vi "tank_auto_sub_straight.vi"(8 "Input Data":i32[](array[numeric]), 10 "Drive Control":T2={"Left X"=0, "Left Y"=0, "Right Y"=0, "Power (100)"=100, "Wait (ms)"=100, "Enc/Deg Target"=0, "Move Type"=enum."Wait"} {"Power (100)" min=-100 max=100}, 11 "NXT/EV3":T1) -> (0 "Output Data":i32[](array[numeric]), 3 "NXT/EV3 out":T1, 4 "Time Out?":bool)   [LabVIEW 2012, in "Serenity_mk2.lvrbt"]
uses:
  Serenity_mk2.lvrbt
  SubVIs/auto_drive_TYP.ctl
  <vilib>/NXT/Subs/LVHSConnector.ctl
  <vilib>/NXT/LegoClasses/BrickReference/BrickReference.lvclass
  <vilib>/FTC/FTC ControllerState.ctl
  <vilib>/FTC/FTC POVState.ctl
  <vilib>/NXT/Hardware/Plugins/Tetrix DC Motor/TetrixDCMotorAddress.ctl
  <vilib>/NXT/HiTechnic/HiTechnic Controls/HiTechnic Port.ctl
  <vilib>/NXT/Block Support/NXT_InputPort.ctl
  <vilib>/FTC/FTC Calculate Drive Power - Tank.vi
  <vilib>/NXT/NXTIO Xnodes/NXTIONodeSubVIs/TETRIX IO Move DC Motors.vi
  <vilib>/NXT/NXTIO Xnodes/NXTIONodeSubVIs/TETRIX IO Motor Status.vi
  <vilib>/NXT/Dual Mode Library/prims/inRangeAndCoerce/inRangeAndCoerce_int8.vi
  <vilib>/NXT/Dual Mode Library/Sound/Tone.vi
  <vilib>/NXT/NXTIO Xnodes/NXTIONodeSubVIs/TETRIX IO Stop DC Motors.vi
  <vilib>/NXT/NXTIO Xnodes/AddressXNode/NXTIOAddress.xnode
  <vilib>/NXT/NXTIO Xnodes/NXTIOXNode/NXTIO.xnode
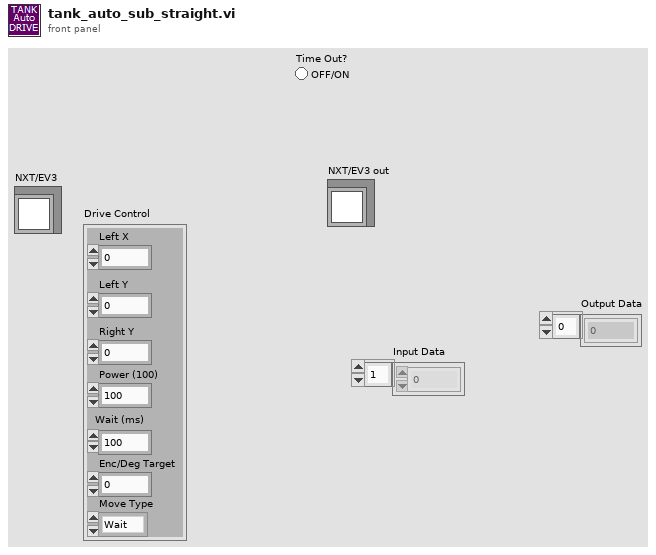
[diagram p1: front panel]
types:
  T1 = typedef "LVHSConnector.ctl" = refnum<class "BrickReference.lvclass">
  T2 = typedef "auto_drive_TYP.ctl" = cluster{"Left X":i8, "Left Y":i8, "Right Y":i8, "Power (100)":i8, "Wait (ms)":u32, "Enc/Deg Target":i32, "Move Type":enum16{"Relative Degrees", "Wait", "Encoder"}}
  T3 = typedef "FTC ControllerState.ctl" = cluster{"Left X":i8, "Left Y":i8, "Right X":i8, "Right Y":i8, "Button Encoding 9-12":u8, "Button Encoding 1-8":u8, "POV":T4}
  T4 = typedef "FTC POVState.ctl" = i8
  T5 = typedef "HiTechnic Port.ctl" = cluster{"Port":T6, "MUX Port":u8}
  T6 = typedef "NXT_InputPort.ctl" = u32
  T7 = typedef "TetrixDCMotorAddress.ctl" = i32
  T8 = cluster{"TetrixDCMotor":T7, "TetrixDCMotor 2":T7}
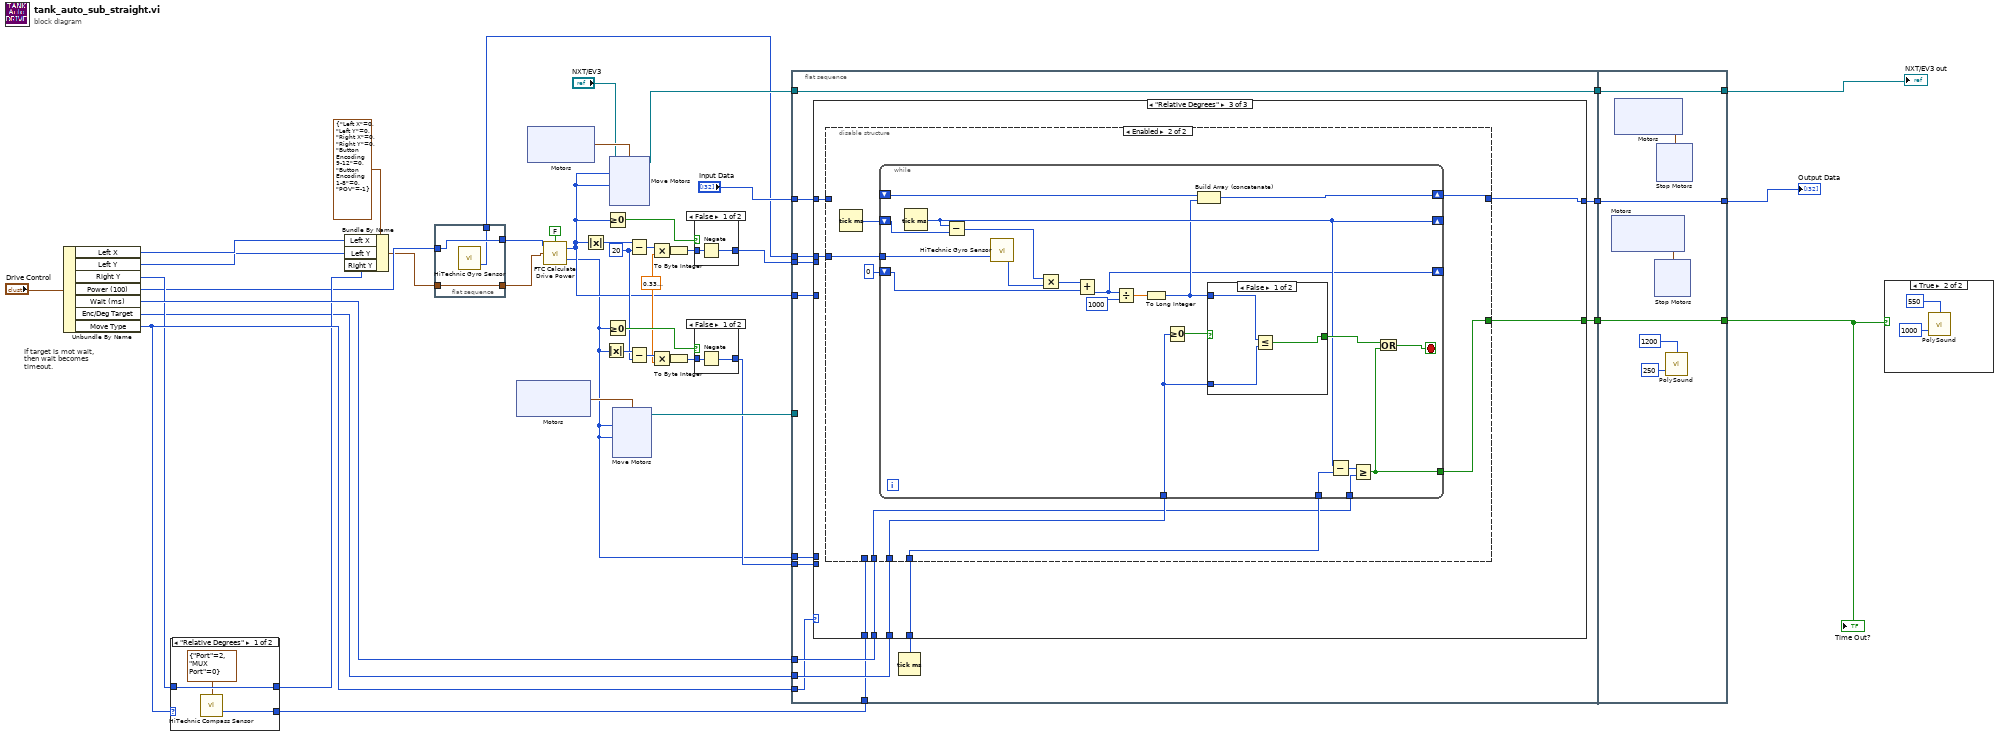
[diagram p0: block diagram]
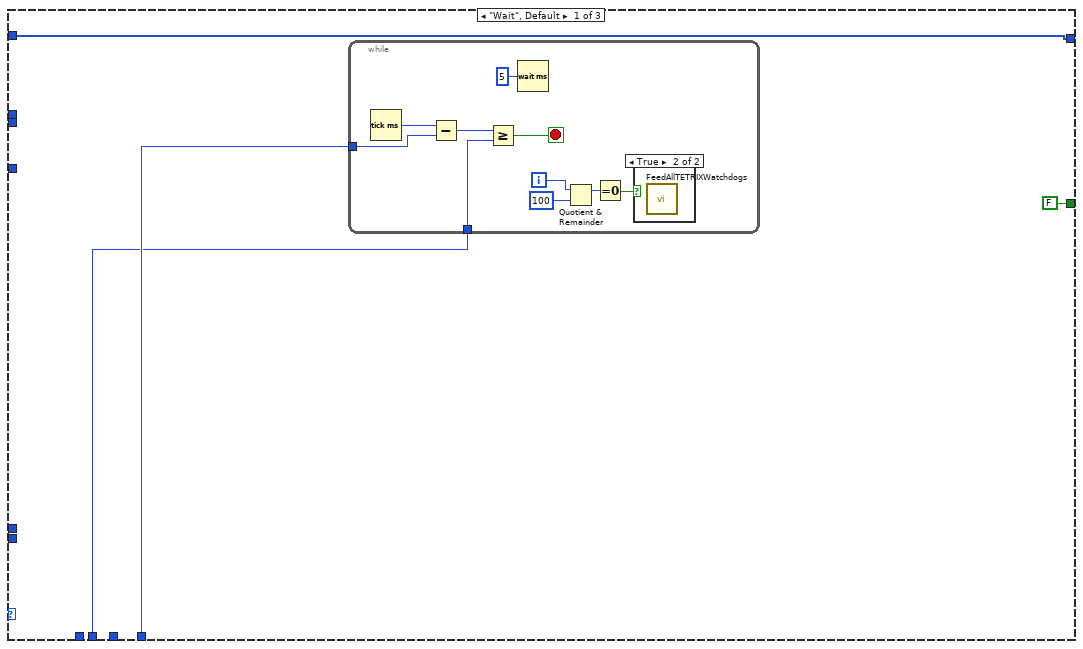
[diagram p6: hidden frame]
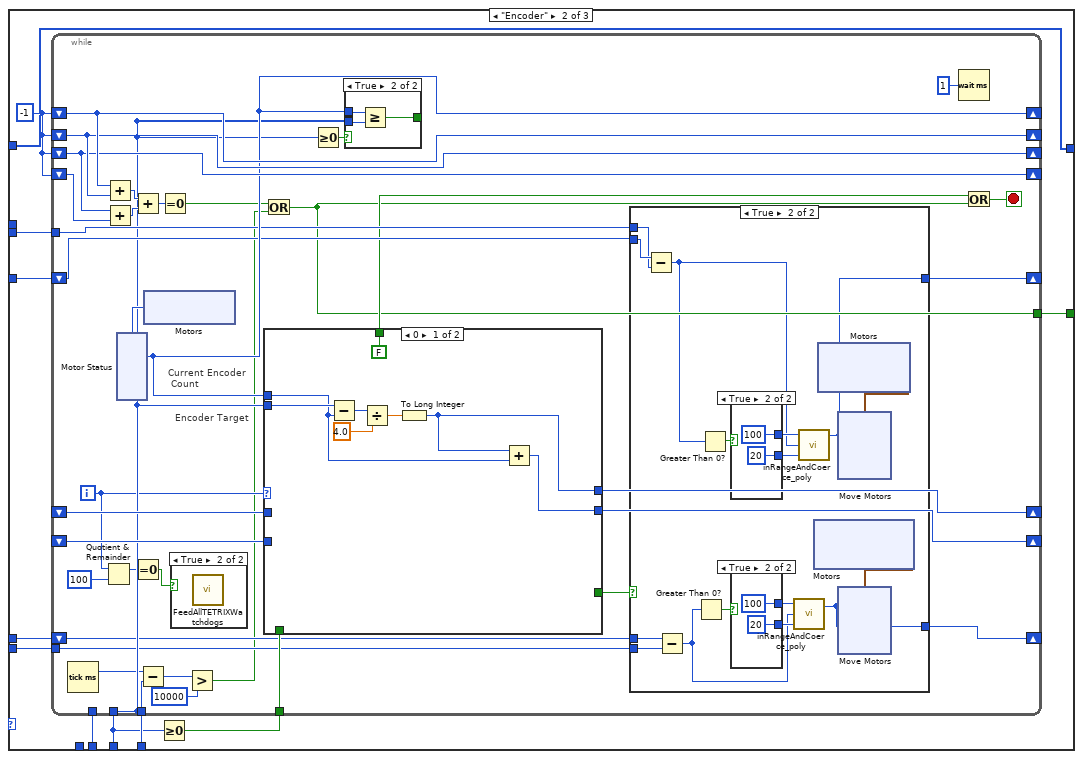
[diagram p8: hidden frame]
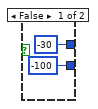
[diagram p11: hidden frame]
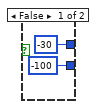
[diagram p12: hidden frame]
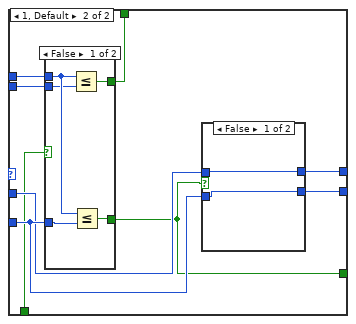
[diagram p13: hidden frame]
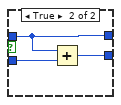
[diagram p14: hidden frame]
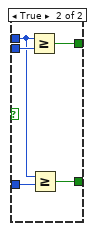
[diagram p15: hidden frame]
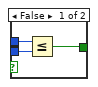
[diagram p16: hidden frame]
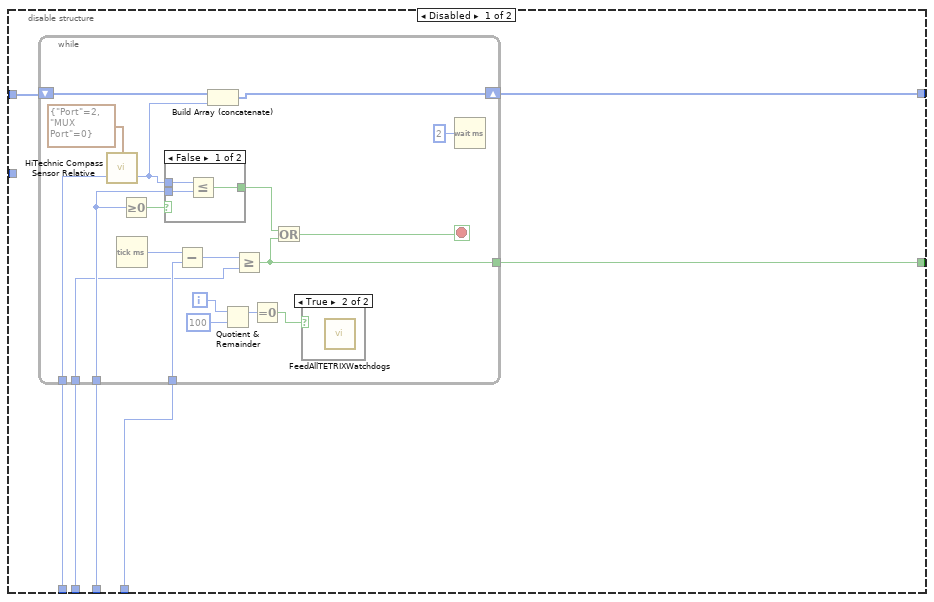
[diagram p17: hidden frame]
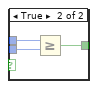
[diagram p19: hidden frame]
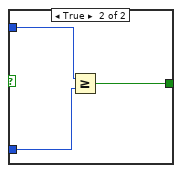
[diagram p20: hidden frame]
diagram:
  w15 = sgl 0.33 ("y")
  w16 = i8 20 ("y")
  # "If target is mot wait, then wait becomes timeout."
  n1 = Unbundle By Name("Drive Control") -> ("Left X"=w38:i8, "Left Y"=w37:i8, "Right Y"=w27:i8, "Power (100)"=w6:i8, "Wait (ms)"=w34:u32, "Enc/Deg Target"=w1:i32, "Move Type"=w29:enum16{"Relative Degrees", "Wait", "Encoder"})
  n2 = case shown="\"Relative Degrees\"" w29 {
    tunnel: [w47 _] -> w2
    tunnel: [w46 w48] -> w28
    tunnel: w27 -> [w46 w48]
    frame "Relative Degrees" {
      n3 = call <vilib>:"HiTechnic Compass Sensor.vi"("Port/MUX"=T5 {"Port"=2, "MUX Port"=0}) -> ("Heading (degrees)"=w47:i16)  [unwired: 2 in, 1 out]
    }
    frame "Wait", Default {
    }
  }
  n4 = Bundle By Name(cluster=T3 {"Left X"=0, "Left Y"=0, "Right X"=0, "Right Y"=0, "Button Encoding 9-12"=0, "Button Encoding 1-8"=0, "POV"=-1} ("Controller State"), "Left X"=w38, "Left Y"=w37, "Right Y"=w28) -> (w4:T3)
  n5 = flat-sequence {
    tunnel: [w51] -> w7
    tunnel: w6 -> [w51]
    tunnel: [w50] -> w5
    tunnel: w4 -> [w50]
    tunnel: [w49] -> w3
    frame #0 {
      n6 = call <vilib>:"HiTechnic Gyro Sensor.vi"() -> ("Gyro Value"=w49:i16)  [unwired: 3 in, 1 out]
    }
  }
  n7 = xnode ("Motors")() -> ("Motor"=w43:cluster{"TetrixDCMotor":T7, "TetrixDCMotor":T7})
  n8 = xnode ("Motors")() -> ("Motor"=w42:cluster{"TetrixDCMotor":T7, "TetrixDCMotor":T7})
  n9 = call-poly <vilib>:"FTC Calculate Drive Power.vi"("Reverse"=FALSE, "Controller State"=w5, "Power Level (50)"=w7) -> ("Right Motor Power"=w11:i8, "Left Motor Power"=w14:i8)  [unwired: 1 in]
  n10 = Absolute Value(x=w14) -> (abs(x)=w26:i8)
  n11 = Absolute Value(x=w11) -> (abs(x)=w17:i8)
  n12 = Greater Or Equal To 0?(x=w14) -> (x >= 0?=w24:bool)
  n13 = Greater Or Equal To 0?(x=w11) -> (x >= 0?=w19:bool)
  n14 = xnode ("Move Motors")("Power/Speed 2"=w14, "Power/Speed 1"=w14, "Motors"=w42, "NXT/EV3"="NXT/EV3") -> ("NXT/EV3"=w36:T1)
  n15 = xnode ("Move Motors")("Power/Speed 2"=w11, "Power/Speed 1"=w11, "Motors"=w43) -> ("NXT/EV3"=w35:T1)  [unwired: 1 in]
  n16 = Subtract(x=w26, y=w16) -> (x-y=w25:i8)
  n17 = Subtract(x=w17, y=w16) -> (x-y=w18:i8)
  n18 = Multiply(x=w25, y=w15) -> (x*y=w23:sgl)
  n19 = Multiply(x=w18, y=w15) -> (x*y=w20:sgl)
  n20 = To Byte Integer(number=w23) -> (8bit integer=w22:i8)
  n21 = To Byte Integer(number=w20) -> (8bit integer=w21:i8)
  n22 = case shown="False" w24 {
    tunnel: w22 -> [w52 w54]
    tunnel: [w53 w54] -> w13
    frame False {
      n23 = Negate(x=w52) -> (-x=w53:i8)
    }
    frame True {
    }
  }
  n24 = case shown="False" w19 {
    tunnel: w21 -> [w55 w57]
    tunnel: [w56 w57] -> w12
    frame False {
      n25 = Negate(x=w55) -> (-x=w56:i8)
    }
    frame True {
    }
  }
  n26 = flat-sequence {
    tunnel: w36 -> [w71]
    tunnel: w35 -> [_]
    tunnel: w34 -> [w70]
    tunnel: [w71] -> w44
    tunnel: w1 -> [w69]
    tunnel: w29 -> [w68]
    tunnel: w2 -> [w67]
    tunnel: [w65] -> w31
    tunnel: w14 -> [w64]
    tunnel: w13 -> [w63]
    tunnel: w12 -> [w62]
    tunnel: w11 -> [w61]
    tunnel: "Input Data" -> [w60]
    tunnel: [w59] -> w8
    tunnel: w3 -> [w58]
    tunnel: [w306] -> w33
    tunnel: w44 -> [w306]
    tunnel: [w303] -> w30
    tunnel: w31 -> [w303]
    tunnel: [w300] -> w9
    tunnel: w8 -> [w300]
    frame #0 {
      n27 = Tick Count (ms)() -> (millisecond timer value=w66:u32)
      n28 = case shown="\"Relative Degrees\"" w68 {
        tunnel: w70 -> [w73 w95 w229]
        tunnel: w69 -> [_ w89 w231]
        tunnel: w67 -> [_ _ w232]
        tunnel: w66 -> [w74 w96 w230]
        tunnel: [FALSE w94 w228] -> w65
        tunnel: w64 -> [_ w92 _]
        tunnel: w63 -> [_ w91 _]
        tunnel: w62 -> [_ w88 _]
        tunnel: w61 -> [_ w87 _]
        tunnel: w60 -> [w72 w86 w227]
        tunnel: [w72 w86 w226] -> w59
        tunnel: w58 -> [_ _ w225]
        frame "Wait", Default {
          n29 = while {
            tunnel: w74 -> [w83]
            tunnel: w73 -> [w82]
            i -> [w77]
            stop <- w81 stop-if-true
            n30 = Tick Count (ms)() -> (millisecond timer value=w85:u32)
            n31 = Subtract(x=w85, y=w83) -> (x-y=w84:u32)
            n32 = Greater Or Equal?(x=w84, y=w82) -> (x >= y?=w81:bool)
            n33 = Wait (ms)(milliseconds to wait=u32 5) -> ()  [unwired: 1 out]
            n34 = Quotient & Remainder(x=w77, y=100) -> (x-y*floor(x/y)=w78:i32)  [unwired: 1 out]
            n35 = Equal To 0?(x=w78) -> (x = 0?=w76:bool)
            n36 = case shown="True" w76 {
              frame False {
              }
              frame True {
                n37 = call <vilib>:"FeedAllTETRIXWatchdogs.vi"() -> ()  [unwired: 11 in, 1 out]
              }
            }
          }
        }
        frame "Encoder" {
          w93 = -1 ("Position 1")
          n38 = Greater Or Equal To 0?(x=w89) -> (x >= 0?=w90:bool)
          n39 = while {
            tunnel: w89 -> [w115]
            tunnel: w96 -> [w102]
            tunnel: w95 -> [_]
            tunnel: [w98] -> w94
            shift-right: [w122] -> _
            shift-left: w93 -> [w126]
            shift-right: [w126] -> _
            shift-left: w93 -> [w125]
            shift-right: [w125] -> _
            shift-left: w93 -> [w124]
            shift-right: [w124] -> _
            shift-left: w93 -> [w127]
            shift-right: [w109] -> _
            shift-left: w92 -> [w121]
            tunnel: w91 -> [w120]
            shift-right: [w118] -> _
            shift-left: _ -> [w119]
            shift-right: [w116] -> _
            shift-left: _ -> [w117]
            tunnel: [w115] -> _
            tunnel: w90 -> [w114]
            tunnel: w88 -> [w111]
            shift-right: [w108] -> _
            shift-left: w87 -> [w110]
            i -> [w107]
            stop <- w131 stop-if-true
            # "Current Encoder\n Count"
            # "Encoder Target"
            n40 = Tick Count (ms)() -> (millisecond timer value=w103:u32)
            n41 = Quotient & Remainder(x=w107, y=100) -> (x-y*floor(x/y)=w105:i32)  [unwired: 1 out]
            n42 = Add(x=w126, y=w125) -> (x+y=w129:i32)
            n43 = Add(x=w124, y=w127) -> (x+y=w128:i32)
            n44 = Add(x=w129, y=w128) -> (x+y=w123:i32)
            n45 = Equal To 0?(x=w105) -> (x = 0?=w104:bool)
            n46 = Subtract(x=w103, y=w102) -> (x-y=w101:u32)
            n47 = xnode "Motors"() -> ("Motor"=w133:T7)
            n48 = xnode "Motor Status"("Motors"=w133) -> ("Position 1"=w122:i32)  [unwired: 1 in, 2 out]
            n49 = Equal To 0?(x=w123) -> (x = 0?=w99:bool)
            n50 = case shown="True" w104 {
              frame False {
              }
              frame True {
                n51 = call <vilib>:"FeedAllTETRIXWatchdogs.vi"() -> ()  [unwired: 11 in, 1 out]
              }
            }
            n52 = Greater?(x=w101, y=u32 10000) -> (0:w97:bool)
            n53 = Or(x=w99, y=w97) -> (x .or. y?=w98:bool)
            n54 = case shown="0" w107 {
              tunnel: w122 -> [w179 w194]
              tunnel: w115 -> [w185 w193]
              tunnel: w119 -> [_ w192]
              tunnel: [w181 w191] -> w118
              tunnel: w117 -> [_ w189]
              tunnel: [w180 w190] -> w116
              tunnel: w114 -> [_ w188]
              tunnel: [_ w187] -> w113
              tunnel: [FALSE w186] -> w112
              frame 0 {
                n55 = Subtract(x=w185, y=w179) -> (x-y=w184:i32)
                n56 = Divide(x=w184, y=sgl 4.0) -> (x/y=w182:sgl)
                n57 = To Long Integer(number=w182) -> (32bit integer=w180:i32)
                n58 = Add(x=w180, y=w179) -> (x+y=w181:i32)
              }
              frame 1, Default {
                n59 = case shown="False" w188 {
                  tunnel: w194 -> [w204 w208]
                  tunnel: w193 -> [w203 w209]
                  tunnel: w192 -> [w200 w207]
                  tunnel: [w202 w206] -> w187
                  tunnel: [w201 w205] -> w186
                  frame False {
                    n60 = Less Or Equal?(x=w204, y=w203) -> (x <= y?=w201:bool)
                    n61 = Less Or Equal?(x=w204, y=w200) -> (x <= y?=w202:bool)
                  }
                  frame True {
                    n62 = Greater Or Equal?(x=w208, y=w209) -> (x >= y?=w205:bool)
                    n63 = Greater Or Equal?(x=w208, y=w207) -> (x >= y?=w206:bool)
                  }
                }
                n64 = case shown="False" w187 {
                  tunnel: w192 -> [w195 w199]
                  tunnel: [w195 w198] -> w191
                  tunnel: [w196 w197] -> w190
                  tunnel: w189 -> [w196 w197]
                  frame False {
                  }
                  frame True {
                    n65 = Add(x=w197, y=w199) -> (x+y=w198:i32)
                  }
                }
              }
            }
            n66 = Greater Or Equal To 0?(x=w115) -> (x >= 0?=w132:bool)
            n67 = case shown="True" w132 {
              tunnel: w115 -> [_ w214]
              tunnel: w122 -> [w212 w215]
              tunnel: [w210 w213] -> _
              tunnel: w115 -> [w211 _]
              frame False {
                n68 = Less Or Equal?(x=w212, y=w211) -> (x <= y?=w210:bool)
              }
              frame True {
                n69 = Greater Or Equal?(x=w215, y=w214) -> (x >= y?=w213:bool)
              }
            }
            n70 = case shown="True" w113 {
              tunnel: w121 -> [w134 w149]
              tunnel: w120 -> [_ w148]
              tunnel: w111 -> [_ w143]
              tunnel: w110 -> [w135 w142]
              tunnel: [w134 w137] -> w109
              tunnel: [w135 w136] -> w108
              frame False {
              }
              frame True {
                n71 = Subtract(x=w149, y=w148) -> (x-y=w144:i8)
                n72 = Subtract(x=w142, y=w143) -> (x-y=w138:i8)
                n73 = Greater Than 0?(x=w138) -> (x > 0?=w139:bool)
                n74 = Greater Than 0?(x=w144) -> (x > 0?=w145:bool)
                n75 = case shown="True" w145 {
                  tunnel: [i8 -30 ("upper limit") i8 100 ("upper limit")] -> w147
                  tunnel: [i8 -100 ("upper limit") i8 20 ("upper limit")] -> w146
                  frame False {
                  }
                  frame True {
                  }
                }
                n76 = case shown="True" w139 {
                  tunnel: [i8 -30 ("upper limit") i8 100 ("upper limit")] -> w141
                  tunnel: [i8 -100 ("upper limit") i8 20 ("upper limit")] -> w140
                  frame False {
                  }
                  frame True {
                  }
                }
                n77 = call-poly <vilib>:"inRangeAndCoerce_poly.vi"("lower limit"=w140, "x"=w138, "upper limit"=w141) -> ("coerced(x)"=w136:i8)  [unwired: 1 out]
                n78 = call-poly <vilib>:"inRangeAndCoerce_poly.vi"("lower limit"=w146, "x"=w144, "upper limit"=w147) -> ("coerced(x)"=w137:i8)  [unwired: 1 out]
                n79 = xnode "Motors"() -> ("Motor"=w150:cluster{"TetrixDCMotor":T7, "TetrixDCMotor":T7})
                n80 = xnode "Motors"() -> ("Motor"=w151:cluster{"TetrixDCMotor":T7, "TetrixDCMotor":T7})
                n81 = xnode ("Move Motors")("Power/Speed 2"=w137, "Power/Speed 1"=w137, "Motors"=w151) -> ()  [unwired: 1 in, 1 out]
                n82 = xnode ("Move Motors")("Power/Speed 2"=w136, "Power/Speed 1"=w136, "Motors"=w150) -> ()  [unwired: 1 in, 1 out]
              }
            }
            n83 = Wait (ms)(milliseconds to wait=u32 1) -> ()  [unwired: 1 out]
            n84 = Or(x=w112, y=w98) -> (x .or. y?=w131:bool)
          }
        }
        frame "Relative Degrees" {
          n85 = disable-structure shown="Enabled" {
            disable-tunnel: w232 -> [w239 _]
            disable-tunnel: w231 -> [w238 w270]
            disable-tunnel: w230 -> [w237 w269]
            disable-tunnel: w229 -> [w236 w268]
            disable-tunnel: [w235 w267] -> w228
            disable-tunnel: w227 -> [w234 _]
            disable-tunnel: [w233 w266] -> w226
            disable-tunnel: w225 -> [_ w271]
            frame Disabled {
              n86 = while {
                tunnel: w239 -> [w257]
                tunnel: w238 -> [w256]
                tunnel: w237 -> [w253]
                tunnel: w236 -> [w251]
                tunnel: [w248] -> w235
                shift-right: [w240] -> w233
                shift-left: w234 -> [w242]
                i -> [w243]
                stop <- w249 stop-if-true
                n87 = call <vilib>:"HiTechnic Compass Sensor Relative.vi"("Target Heading (Degrees)"=w257, "Port/MUX"=T5 {"Port"=2, "MUX Port"=0}) -> ("Relative Heading (Degrees)"=w241:i32)  [unwired: 1 in, 1 out]
                n88 = Tick Count (ms)() -> (millisecond timer value=w254:u32)
                n89 = Greater Or Equal To 0?(x=w256) -> (x >= 0?=w255:bool)
                n90 = case shown="False" w255 {
                  tunnel: w256 -> [w259 w264]
                  tunnel: [w261 w263] -> w250
                  tunnel: w241 -> [w260 w262]
                  frame False {
                    n91 = Less Or Equal?(x=w260, y=w259) -> (x <= y?=w261:bool)
                  }
                  frame True {
                    n92 = Greater Or Equal?(x=w262, y=w264) -> (x >= y?=w263:bool)
                  }
                }
                n93 = Subtract(x=w254, y=w253) -> (x-y=w252:u32)
                n94 = Build Array (concatenate)(w242, w241) -> (w240:i32[])
                n95 = Quotient & Remainder(x=w243, y=100) -> (x-y*floor(x/y)=w245:i32)  [unwired: 1 out]
                n96 = Greater Or Equal?(x=w252, y=w251) -> (x >= y?=w248:bool)
                n97 = Equal To 0?(x=w245) -> (x = 0?=w244:bool)
                n98 = Or(x=w250, y=w248) -> (x .or. y?=w249:bool)
                n99 = case shown="True" w244 {
                  frame False {
                  }
                  frame True {
                    n100 = call <vilib>:"FeedAllTETRIXWatchdogs.vi"() -> ()  [unwired: 11 in, 1 out]
                  }
                }
                n101 = Wait (ms)(milliseconds to wait=u32 2) -> ()  [unwired: 1 out]
              }
            }
            frame Enabled {
              n102 = Tick Count (ms)() -> (millisecond timer value=w272:u32)
              n103 = while {
                shift-right: [w283] -> _
                shift-left: w272 -> [w275]
                tunnel: w271 -> [w290]
                tunnel: w270 -> [w287]
                tunnel: w269 -> [w284]
                tunnel: w268 -> [w281]
                tunnel: [w280] -> w267
                shift-right: [w277] -> w266
                shift-left: _ -> [w278]
                shift-right: [w274] -> _
                shift-left: u32 0 -> [w273]
                stop <- w285 stop-if-true
                n104 = Tick Count (ms)() -> (millisecond timer value=w283:u32)
                n105 = Subtract(x=w283, y=w275) -> (x-y=w289:u32)
                n106 = call <vilib>:"HiTechnic Gyro Sensor.vi"("Offset"=w290) -> ("Gyro Value"=w293:i16)  [unwired: 2 in, 1 out]
                n107 = Multiply(x=w289, y=w293) -> (x*y=w292:u32)
                n108 = Add(x=w292, y=w273) -> (x+y=w274:u32)
                n109 = Divide(x=w274, y=1000) -> (x/y=w279:dbl)
                n110 = To Long Integer(number=w279) -> (32bit integer=w276:i32)
                n111 = Greater Or Equal To 0?(x=w287) -> (x >= 0?=w288:bool)
                n112 = Build Array (concatenate)(w278, w276) -> (w277:i32[])
                n113 = case shown="False" w288 {
                  tunnel: w287 -> [w295 w298]
                  tunnel: w276 -> [w296 w299]
                  tunnel: [w294 w297] -> w286
                  frame False {
                    n114 = Less Or Equal?(x=w296, y=w295) -> (x <= y?=w294:bool)
                  }
                  frame True {
                    n115 = Greater Or Equal?(x=w299, y=w298) -> (x >= y?=w297:bool)
                  }
                }
                n116 = Subtract(x=w283, y=w284) -> (x-y=w282:u32)
                n117 = Greater Or Equal?(x=w282, y=w281) -> (x >= y?=w280:bool)
                n118 = Or(x=w286, y=w280) -> (x .or. y?=w285:bool)
              }
            }
          }
        }
      }
    }
    frame #1 {
      n119 = xnode "Motors"() -> ("Motor"=w304:cluster{"TetrixDCMotor":T7, "TetrixDCMotor":T7})
      n120 = xnode "Motors"() -> ("Motor"=w305:cluster{"TetrixDCMotor":T7, "TetrixDCMotor":T7})
      n121 = xnode "Stop Motors"("Motors"=w304) -> ()  [unwired: 1 in, 1 out]
      n122 = xnode "Stop Motors"("Motors"=w305) -> ()  [unwired: 1 in, 1 out]
      n123 = call-poly <vilib>:"PolySound.vi"("Duration (500 ms)"=u16 250, "Tone (440 Hz)"=u16 1200) -> ()  [unwired: 2 in, 1 out]
    }
  }
  n124 = case shown="True" w30 {
    frame False {
    }
    frame True {
      n125 = call-poly <vilib>:"PolySound.vi"("Duration (500 ms)"=u16 1000, "Tone (440 Hz)"=u16 550) -> ()  [unwired: 2 in, 1 out]
    }
  }
  "NXT/EV3 out" <- w33
  "Time Out?" <- w30
  "Output Data" <- w9
